vi "Pre Launch Init.vi"(11 "Series UI Actor in":refnum<class "Series UI Actor.lvclass">) -> (0 "error out":errorcluster, 3 "Series UI Actor out":refnum<class "Series UI Actor.lvclass">)   [LabVIEW 2024, in "Series UI Actor.lvlib" / "Series UI Actor.lvclass"]
doc: "Initializes the panel actor. Creates the Panel Helper.\n\n----\nPlease see the following web address for additional documentation and tutorial information:\nhttp://www.mooregoodideas.com/mgi-panel-manager/\n\nAuthor: Derek Trepanier\n\nCopyright (c) 2018, Moore Good Ideas, Inc.\n\nAll rights reserved.\n\nRedistribution and use in source and binary forms, with or without modification, are permitted provided that the following conditions are met:\n\n * Redistributions of source code must retain the above copyright notice, this list of conditions and the following disclaimer.\n * Redistributions in binary form must reproduce the above copyright notice, this list of conditions and the following disclaimer in the documentation and/or other materials provided with the distribution.\n * Neither the name of Moore Good Ideas, Inc. nor the names of its contributors may be used to endorse or promote products derived from this software without specific prior written permission.\n\nTHIS SOFTWARE IS PROVIDED BY THE COPYRIGHT HOLDERS AND CONTRIBUTORS \"AS IS\" AND ANY EXPRESS OR IMPLIED WARRANTIES, INCLUDING, BUT NOT LIMITED TO, THE IMPLIED WARRANTIES OF MERCHANTABILITY AND FITNESS FOR A PARTICULAR PURPOSE ARE DISCLAIMED. IN NO EVENT SHALL THE COPYRIGHT OWNER OR CONTRIBUTORS BE LIABLE FOR ANY DIRECT, INDIRECT, INCIDENTAL, SPECIAL, EXEMPLARY, OR CONSEQUENTIAL DAMAGES (INCLUDING, BUT NOT LIMITED TO, PROCUREMENT OF SUBSTITUTE GOODS OR SERVICES; LOSS OF USE, DATA, OR PROFITS; OR BUSINESS INTERRUPTION) HOWEVER CAUSED AND ON ANY THEORY OF LIABILITY, WHETHER IN CONTRACT, STRICT LIABILITY, OR TORT (INCLUDING NEGLIGENCE OR OTHERWISE) ARISING IN ANY WAY OUT OF THE USE OF THIS SOFTWARE, EVEN IF ADVISED OF THE POSSIBILITY OF SUCH DAMAGE."
uses:
  Series UI Actor.lvclass
  Series UI Actor.lvclass/Series UI Actor.ctl
  <vilib>/MGI/Panel Manager/Panel Actor/Panel Actor/Panel Actor.lvclass
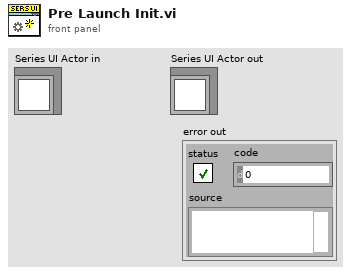
[diagram p1: front panel]
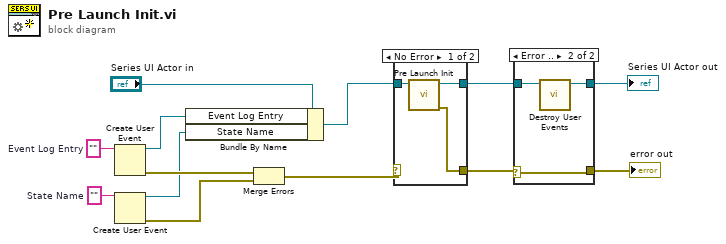
[diagram p0: block diagram]
diagram:
  w4 = ""  # State Name
  w13 = ""  # Event Log Entry
  n1 = Create User Event(user event datatype=w13) -> (user event=w12:refnum<user-event>, error out=w9:errorcluster)  [unwired: 1 in]
  n2 = Create User Event(user event datatype=w4) -> (user event=w3:refnum<user-event>, error out=w1:errorcluster)  [unwired: 1 in]
  n3 = Bundle By Name(cluster="Series UI Actor in", "Event Log Entry"=w12, "State Name"=w3) -> (w11:refnum<class "Series UI Actor.lvclass">)
  n4 = Merge Errors(w9, w1) -> (w2:errorcluster)
  n5 = case shown="No Error" w2 {
    selector: w2 -> [_ w17]
    tunnel: w11 -> [w16 w18]
    tunnel: [w15 w18] -> w10
    tunnel: [w14 w17] -> w8
    frame No Error {
      n6 = call-parent "Pre Launch Init.vi"("Panel Actor in"=w16) -> ("error out"=w14:errorcluster, "Panel Actor out"=w15:refnum<class "Series UI Actor.lvclass">)  [unwired: 9 in]
    }
    frame Error {
    }
  }
  n7 = case shown="Error .." w8 {
    selector: w8 -> [w19 w21]
    tunnel: w10 -> [w20 w23]
    tunnel: [w20 w22] -> w6
    tunnel: [w19 w21] -> w7
    frame No Error {
    }
    frame Error {
      n8 = call "Destroy User Events.vi"("Series UI Actor in"=w23) -> ("Series UI Actor out"=w22:refnum<class "Series UI Actor.lvclass">)  [unwired: 10 in]
    }
  }
  "error out" <- w7
  "Series UI Actor out" <- w6
